vi "Write Device Enqueuer.vi"(8 "error in (no error)":errorcluster, 10 "Device Enqueuer":refnum<class "Message Enqueuer.lvclass">, 11 "CS++DeviceGUIActor in":refnum<class "CS++DeviceGUIActor.lvclass">) -> (0 "error out":errorcluster, 3 "CS++DeviceGUIActor out":refnum<class "CS++DeviceGUIActor.lvclass">)   [LabVIEW 2012, in "CS++DeviceGUIActor.lvlib" / "CS++DeviceGUIActor.lvclass"]
doc: "Write device enqueuer."
uses:
  CS++DeviceGUIActor.lvclass
  <vilib>/ActorFramework/Message Enqueuer/Message Enqueuer.lvclass
  CS++DeviceGUIActor.lvclass/CS++DeviceGUIActor.ctl
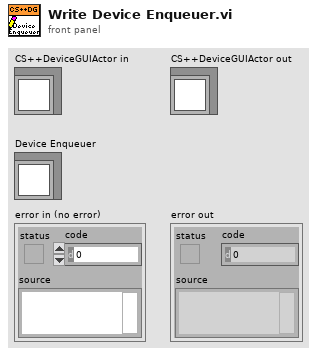
[diagram p1: front panel]
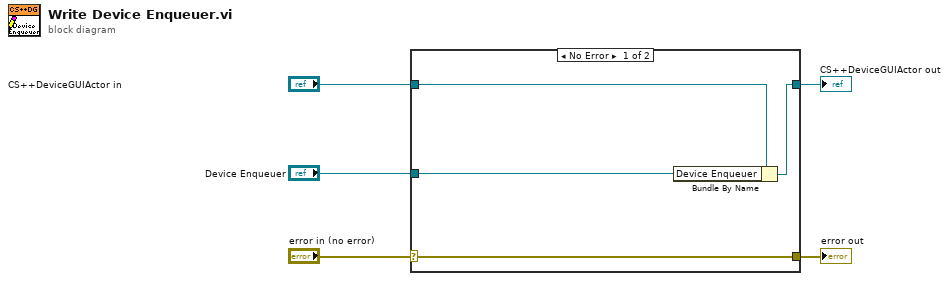
[diagram p0: block diagram]
diagram:
  n1 = case shown="No Error" "error in (no error)" {
    selector: "error in (no error)" -> [w9 w10]
    tunnel: [w9 w10] -> w4
    tunnel: [w7 w11] -> w2
    tunnel: "CS++DeviceGUIActor in" -> [w8 w11]
    tunnel: "Device Enqueuer" -> [w6 _]
    frame No Error {
      n2 = Bundle By Name(cluster=w8, "Device Enqueuer"=w6) -> (w7:refnum<class "CS++DeviceGUIActor.lvclass">)
    }
    frame Error {
    }
  }
  "error out" <- w4
  "CS++DeviceGUIActor out" <- w2
